vi "LEBITVacuum.constructor.vi"(0 "name":string, 2 "data in":string, 5 "error in(no error)":errorcluster) -> (14 "i ref out":refnum<vi>, 16 "data out":string, 19 "error out":errorcluster)   [LabVIEW 2014, in "LEBITVacuum.lvlib"]
doc: "This is the constructor of a class.\n\nLicense Agreement for this software:\n\nCopyright (C)\nGesellschaft für Schwerionenforschung, GSI\nPlanckstr. 1\n64291 Darmstadt\nGermany\n\nContact: D.Beck@gsi.de \n\nThis program is free software; you can redistribute it and/or modify it under the terms of the \nGNU General Public License as published by the Free Software Foundation; either version 2 of \nthe license, or (at your option) any later version.\n\nThis program is distributed in the hope that it will be useful, but WITHOUT ANY WARRANTY; \nwithout even the implied warranty of MERCHANTABILITY or FITNESS FOR A PARTICULAR PURPOSE. See the GNU General License for more details (http://www.gnu.org).\n\nGesellschaft für Schwerionenforschung, GSI\nPlanckstr. 1, 64291 Darmstadt, Germany\nFor all questions and ideas contact: M.Richter@gsi.de, H.Brand@gsi.de or D.Beck@gsi.de.\nLast update: 16-JUN-2004"
uses:
  LEBITVacuum.lvlib
  CSCore/BaseProcess/BaseProcess.lvlib
  CSCore/CSSystem/CSSystemLib/CSSystemLib.lvlib
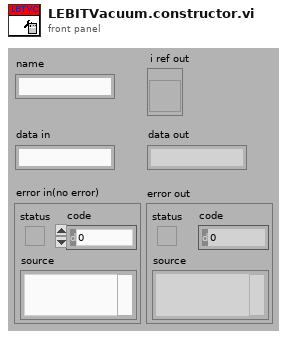
[diagram p1: front panel]
types:
  T1 = enum16{"SetAttribute", "GetAttribute", "CreateAttribute", "DestroyAttribute", "DestroyAllAtributes"}
  T2 = typedef "BaseProcess.lvlib/BaseProcess.i attribute.ctl" = cluster{"EventStatus":string, "EventError":i32, "PresetEvtWatchD":i32, "PresetPdcWatchD":i32, "EventTimeout":i32, "PeriodicInterval":i32, "Interface":string[], "Address":string[], "Special":string[], "PeriodicError":i32, "PeriodicStatus":string, "SuperProc":string, "Descriptors":T3[], "CaseRef":refnum<vi>, "PdcRef":refnum<vi>, "Thread Ref":refnum<vi>, "eventErrorID":i32, "eventStatusID":i32, "periodicErrorID":i32, "periodicStatusID":i32, "pdcCtrID":i32}
  T3 = typedef "BaseProcess.lvlib/BaseProcess.descriptor definition.ctl" = cluster{"selector":string, "descriptor":T4}
  T4 = typedef "BaseProcess.lvlib/BaseProcess.descriptor string definition.ctl" = string
  T5 = typedef "LEBITVacuum.lvlib/LEBITVacuum.i attribute.ctl" = cluster{"setValuePLC":string[], "nickNames":string[], "setValuePLCServiceID":i32[], "monValuePLC":string[], "SetValueServiceID":i32[], "MonValueServiceID":i32[], "SetValue":i16[], "AllPLCValues":string[], "CondSpecial2DArray":string[][], "CondSpecialIndex":i32[], "ReasonForLocking":string, "ReasonForLockingID":i32, "enableValuePLC":string[], "OverwriteCloseSafetyPLC":string[], "OverwriteOpenSafetyPLC":string[], "OverwriteCloseSafetyPLCServiceID":i32[], "OverwriteOpenSafetyPLCServiceID":i32[], "MKS Address Array":i32[][], "MKS MeasurementServiceID":i32[], "MKS Measurement":string[], "CRYO Measurement":string[][], "CRYO MeasurementServiceID":i32[], "Special":string[], "Start Date":string, "MKS VISA resource":refnum<visa-resource-name>, "CRYO VISA resource":refnum<visa-resource-name>}
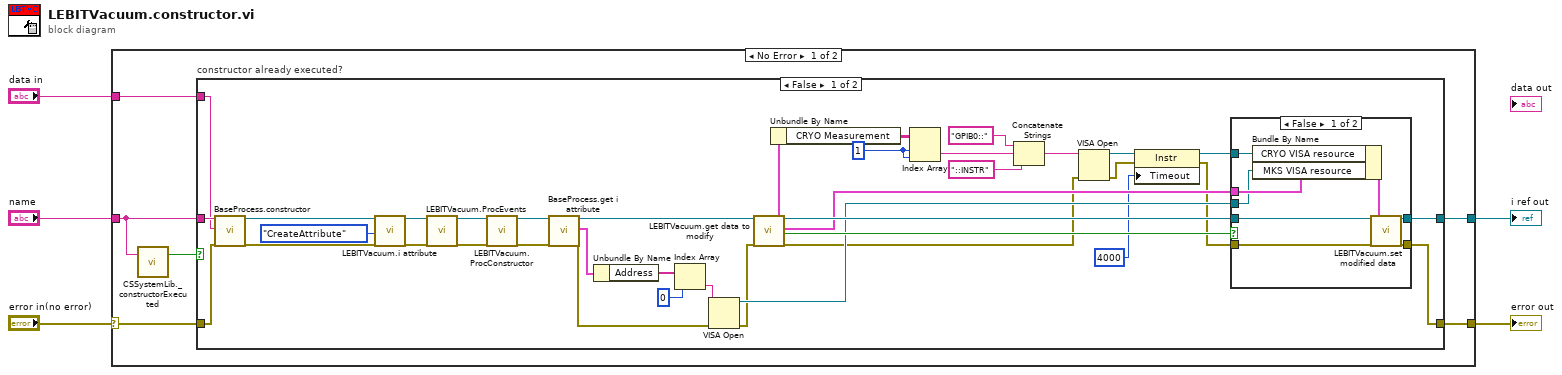
[diagram p0: block diagram]
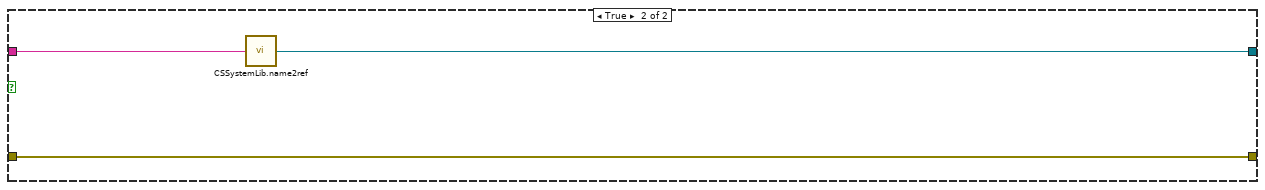
[diagram p3: hidden frame]
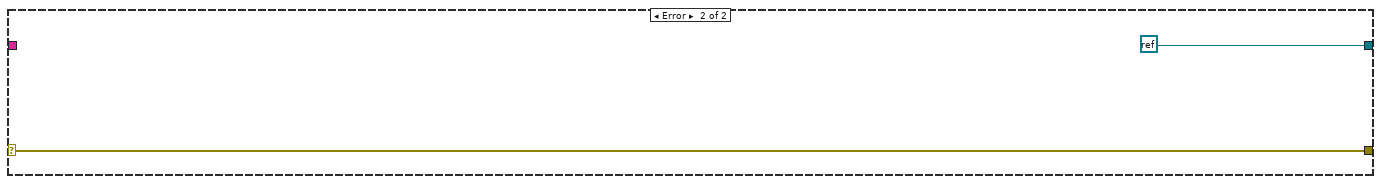
[diagram p4: hidden frame]
diagram:
  n1 = case shown="No Error" "error in(no error)" {
    selector: "error in(no error)" -> [w9 w62]
    tunnel: "name" -> [w8 _]
    tunnel: [w11 refnum<k0> refnum] -> w4
    tunnel: [w10 w62] -> w3
    tunnel: "data in" -> [w6 _]
    frame No Error {
      n2 = call "CSSystemLib._constructorExecuted.vi"("name"=w8) -> ("constructor executed?"=w7:bool)  [unwired: 18 in]
      n3 = case "constructor already executed?" shown="False" w7 {
        tunnel: [w31 w60] -> w11
        tunnel: [w30 w59] -> w10
        tunnel: w9 -> [w44 w59]
        tunnel: w8 -> [w43 w61]
        tunnel: w6 -> [w42 _]
        frame False {
          w22 = 1 ("index (row)")
          n4 = call "BaseProcess.constructor.vi"("name"=w43, "data in"=w42, "error in (no error)"=w44) -> ("i ref out"=w48:refnum<vi>, "error out"=w47:errorcluster)  [unwired: 14 in, 1 out]
          n5 = call "LEBITVacuum.i attribute.vi"("VI Refnum"=w48, "Action"=T1."CreateAttribute", "error in (no error)"=w47) -> ("VI Refnum out"=w46:refnum<vi>, "error out"=w45:errorcluster)  [unwired: 14 in, 1 out]
          n6 = call "LEBITVacuum.ProcEvents.vi"("i ref in"=w46, "error in"=w45) -> ("i ref out"=w40:refnum<vi>, "error out"=w39:errorcluster)  [unwired: 16 in]
          n7 = call "LEBITVacuum.ProcConstructor.vi"("i ref in"=w40, "error in(no error)"=w39) -> ("i ref out"=w37:refnum<vi>, "error out"=w38:errorcluster)  [unwired: 16 in]
          n8 = call "BaseProcess.get i attribute.vi"("i ref in"=w37, "error in (no error)"=w38) -> ("i ref out"=w33:refnum<vi>, "i attribute"=w36:T2, "error out"=w26:errorcluster)  [unwired: 15 in]
          n9 = Unbundle By Name(w36) -> ("Address"=w35:string[])
          n10 = Index Array(array=w35, index=0) -> (element=w28:string)
          n11 = VISA Open(error in (no error)=w26, VISA resource name=w28) -> (VISA resource name=w27:refnum<visa-resource-name>, error out=w25:errorcluster)  [unwired: 3 in]
          n12 = call "LEBITVacuum.get data to modify.vi"("i ref in"=w33, "error in (no error)"=w25) -> ("i ref out"=w32:refnum<vi>, "i attribute"=w24:T5, "timed out"=w29:bool, "error out"=w18:errorcluster)  [unwired: 14 in]
          n13 = Unbundle By Name(w24) -> ("CRYO Measurement"=w23:string[][])
          n14 = Index Array(array=w23, index (row)=w22, index (col)=w22) -> (element=w20:string)
          n15 = Concatenate Strings("GPIB0::" ("string"), w20, "::INSTR" ("string")) -> (w17:string)
          n16 = VISA Open(error in (no error)=w18, VISA resource name=w17) -> (VISA resource name=w16:refnum<visa-resource-name>, error out=w14:errorcluster)  [unwired: 3 in]
          n17 = property class="Instr"(reference=w16, error in=w14, "Timeout"=u32 4000 ("General Settings:Timeout Value")) -> (reference out=w15:refnum<visa-resource-name>, error out=w13:errorcluster)
          n18 = case shown="False" w29 {
            tunnel: w32 -> [w56 w58]
            tunnel: w13 -> [w55 w57]
            tunnel: [w54 w58] -> w31
            tunnel: [w53 w57] -> w30
            tunnel: w24 -> [w52 _]
            tunnel: w27 -> [w50 _]
            tunnel: w15 -> [w49 _]
            frame False {
              n19 = Bundle By Name(cluster=w52, "CRYO VISA resource"=w49, "MKS VISA resource"=w50) -> (w51:T5)
              n20 = call "LEBITVacuum.set modified data.vi"("i ref in"=w56, "i attribute"=w51, "error in (no error)"=w55) -> ("i ref out"=w54:refnum<vi>, "error out"=w53:errorcluster)  [unwired: 15 in]
            }
            frame True {
            }
          }
        }
        frame True {
          n21 = call "CSSystemLib.name2ref.vi"("name"=w61) -> ("obj refnum"=w60:refnum<vi>)
        }
      }
    }
    frame Error {
    }
  }
  "i ref out" <- w4
  "error out" <- w3
